vi "Impedance_Single.vi"(0 "Test Params Cluster":T2={"Test Freq. (Hz)"=25000.0, "Output Signal Amplitude\nVolts Pk"=0.1, "Sampling Time (s)"=0.01, "Sampling Rate (Hz)"=250000.0, "Output Channel"="PXI1Slot2/ao1", "Current Channel"="PXI1Slot2/ai1", "Voltage Channel"="PXI1Slot2/ai0", "Trigger Channel"="/PXI1Slot2/ao/StartTrigger", "Number of runs"=5}, 2 "SaveFile?":bool, 5 "LCR Params":T1={"Rg_Vmon"=5000.0, "Rg_Imon"=5000.0, "ESL_Cal"=2.95e-07, "ESR_Cal"=0.0, "Cp_Cal"=0.0, "Rp_Cal"=1000000000.0, "UseCorrection"=TRUE, "R_Shunt"=100.0} {"R_Shunt" format="%#_6p"; "Rg_Vmon" format="%#_6p"; "Rg_Imon" format="%#_6p"; "ESL_Cal" format="%#_6p"; "ESR_Cal" format="%#_6p"; "Cp_Cal" format="%#_6p"; "Rp_Cal" format="%#_6p"}, 12 "File Name String":string="Test", 13 "Path":path=path "C:/Users/MPI/Documents/Test Saving Data", 14 "Experiment Title":string="Experiment Title") -> (4 "Mean Signal\nImpedance cluster":T3={"|Z|"=131.4492234563314, "Phase(Z)"=77.90762243322018, "Re(Z)"=27.537098036686675, "Imag(Z)"=128.53251175866149, "Ls"=0.0008182633837763256, "Cs"=-4.952986319624157e-08, "Rp"=0.0, "Cp"=0.0} {"|Z|" format="%#_6p"; "Phase(Z)" format="%#_6p"; "Re(Z)" format="%#_6p"; "Imag(Z)" format="%#_6p"; "Ls" format="%#_6p"; "Cs" format="%#_6p"; "Rp" format="%#_6p"; "Cp" format="%#_6p"})   [LabVIEW 2020]
uses:
  <vilib>/Analysis/baseanly.llb/Mean (CDB).vi
  <vilib>/Analysis/NI_AALBase.lvlib
panel:
  out "Progress":i32(slide) scale=0.0..100.0
  in  "Tab Control":enum32{"Inputs", "Outputs", "Additional Plots"}(tab)
  out "Impedance (Mag)":dbl=131.44922360893165 format="%_4p"
  out "Impedance (Phase)":dbl=77.90762242326527 format="%_3p"
  out "Inductance":dbl=0.0008182633837921632 format="%#_3p"
  out "Capacitance":dbl=-4.9529863304224986e-08 format="%#_3p"
  out "Real (Z)":dbl=27.53709808707976 format="%#_4p"
  out "St. Dev - |Z|":dbl=0.006733204606830156 format="%.4p"
  out "St. Dev - L":dbl=4.20379350558212e-08 format="%.2p"
  out "St. Dev - C":dbl=2.5446531556775277e-12 format="%.2p"
  out "St. Dev - R":dbl=0.00676584259927313 format="%.2p"
  out "Mag Real Imag":cluster{"mean":dbl, "mean":dbl, "Imag(Z)":dbl}(graph)
  out "Time domain Voltage":waveform(dbl)(graph)={"t0"=timestamp(3724414950.391881 s since 1904-01-01), "dt"=3.999999999999989e-06, "Y"=array[2500 elements], "attributes"=variant("NI_ChannelName"=variant(string "Dev3/ai0"), "NI_UnitDescription"=variant(string "Volts"))}
  out "Time domain Current\n(Measured Voltage)":waveform(dbl)(graph)={"t0"=timestamp(3724414950.478328 s since 1904-01-01), "dt"=3.999999999999989e-06, "Y"=array[2500 elements], "attributes"=variant("NI_ChannelName"=variant(string "Dev3/ai1"), "NI_UnitDescription"=variant(string "Volts"))}
  out "Inductance 2":dbl(graph)
  out "Current Run #":i32=4
  out "Time domain Signals":waveform(dbl)[](graph)=[{"t0"=timestamp(3724414950.391881 s since 1904-01-01), "dt"=3.999999999999989e-06, "Y"=array[2500 elements], "attributes"=variant("NI_ChannelName"=variant(string "Dev3/ai0"), "NI_UnitDescription"=variant(string "Volts"))}, {"t0"=timestamp(3724414950.478328 s since 1904-01-01), "dt"=3.999999999999989e-06, "Y"=array[2500 elements], "attributes"=variant("NI_ChannelName"=variant(string "Dev3/ai1"), "NI_UnitDescription"=variant(string "Volts"))}]
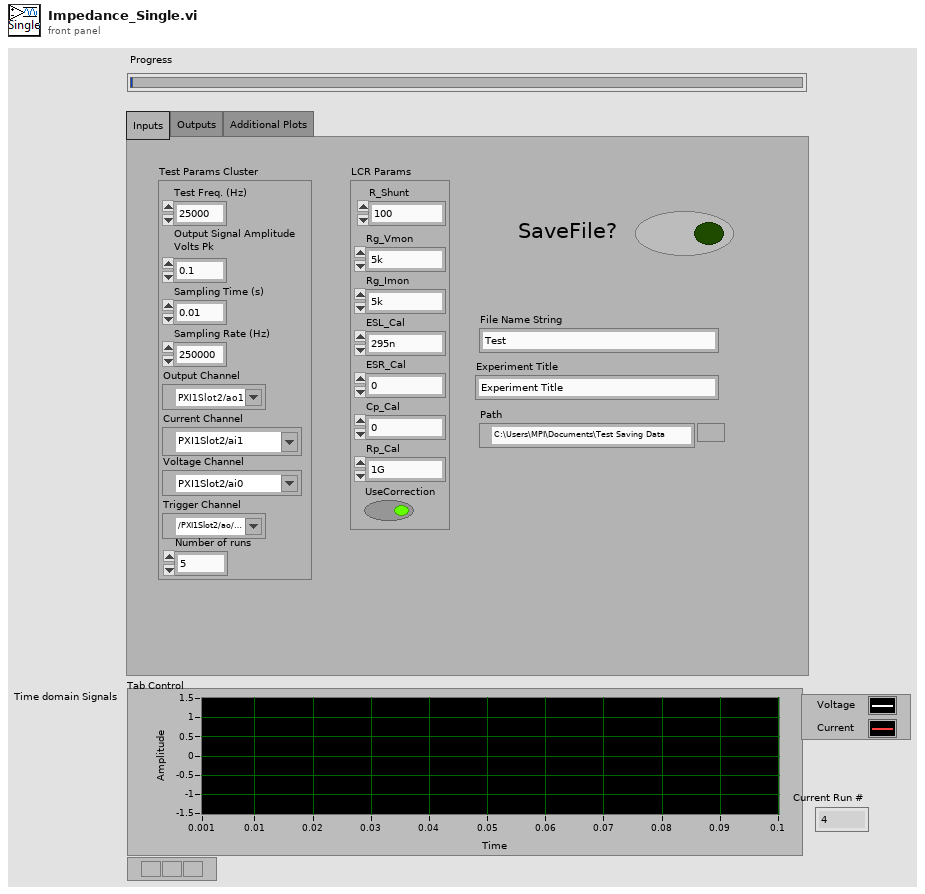
[diagram p1: front panel]
types:
  T1 = cluster{"Rg_Vmon":dbl, "Rg_Imon":dbl, "ESL_Cal":dbl, "ESR_Cal":dbl, "Cp_Cal":dbl, "Rp_Cal":dbl, "UseCorrection":bool, "R_Shunt":dbl}
  T2 = cluster{"Test Freq. (Hz)":dbl, "Output Signal Amplitude\nVolts Pk":dbl, "Sampling Time (s)":dbl, "Sampling Rate (Hz)":dbl, "Output Channel":tag, "Current Channel":tag, "Voltage Channel":tag, "Trigger Channel":tag, "Number of runs":i32}
  T3 = cluster{"|Z|":dbl, "Phase(Z)":dbl, "Re(Z)":dbl, "Imag(Z)":dbl, "Ls":dbl, "Cs":dbl, "Rp":dbl, "Cp":dbl}
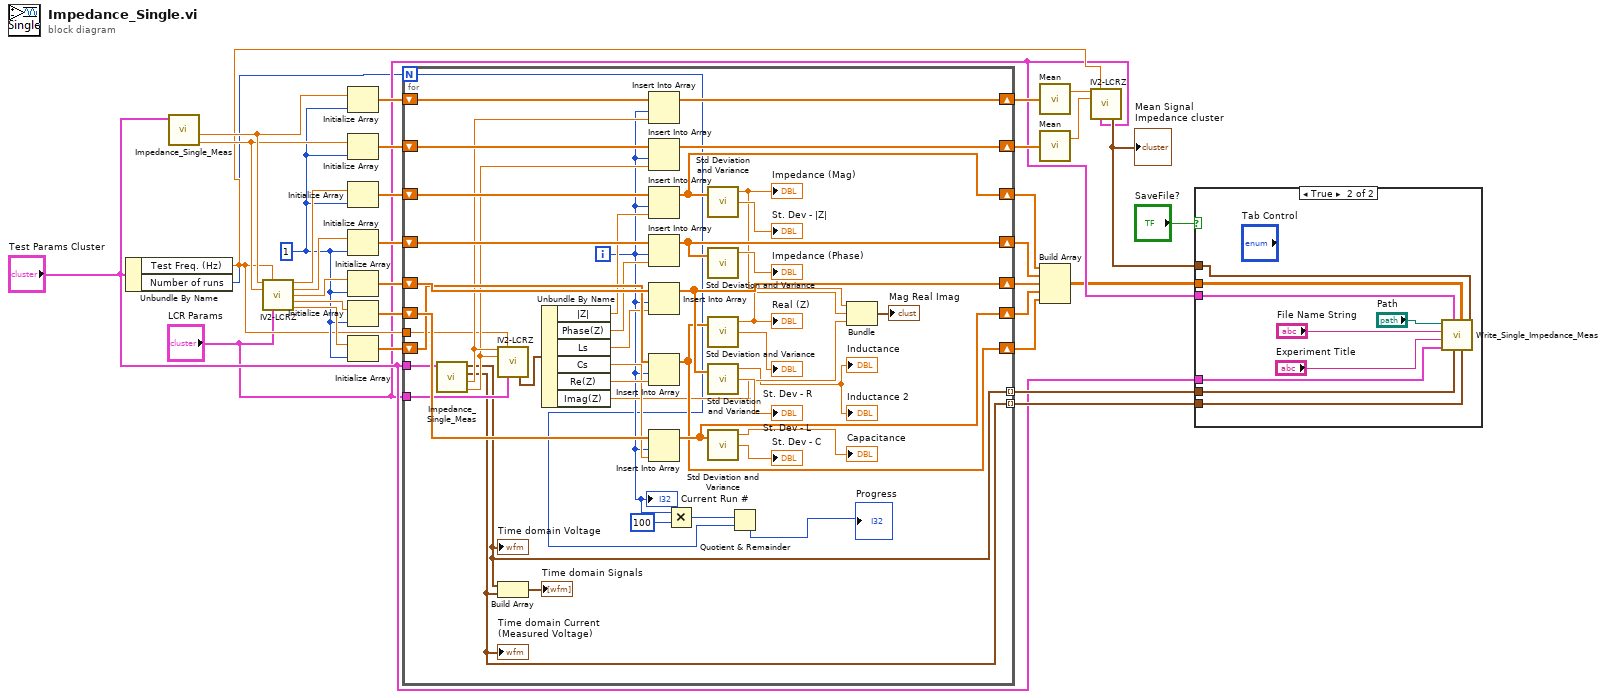
[diagram p0: block diagram]
diagram:
  w21 = 1 ("dimension size")
  n1 = Unbundle By Name("Test Params Cluster") -> ("Test Freq. (Hz)"=w9:dbl, "Number of runs"=w7:i32)
  n2 = call "Impedance_Single_Meas.vi"("Test Params Cluster"="Test Params Cluster") -> ("Current Complex"=w22:cdb, "Voltage Complex"=w23:cdb)  [unwired: 7 in, 2 out]
  n3 = call "IV2-LCRZ.vi"("Voltage In"=w23, "Test Frequency"=w9, "Current In"=w22, "LCR Params"="LCR Params") -> ("Impedance (Mag)"=w31:dbl, "Impedance (Phase)"=w30:dbl, "Ls"=w29:dbl, "Cs"=w28:dbl, "Real (Z)"=w27:dbl)  [unwired: 6 in, 1 out]
  n4 = Initialize Array(w23, w21) -> (w20:cdb[])
  n5 = Initialize Array(w22, w21) -> (w19:cdb[])
  n6 = Initialize Array(w31, w21) -> (w33:dbl[])
  n7 = Initialize Array(w30, w21) -> (w32:dbl[])
  n8 = Initialize Array(w29, w21) -> (w26:dbl[])
  n9 = Initialize Array(w28, w21) -> (w25:dbl[])
  n10 = Initialize Array(w27, w21) -> (w24:dbl[])
  n11 = for {
    N: w7 -> [w34]
    shift-right: [w63] -> w6
    shift-left: w33 -> [w76]
    shift-right: [w62] -> w5
    shift-left: w32 -> [w75]
    shift-right: [w61] -> w4
    shift-left: w26 -> [w74]
    shift-right: [w57] -> w3
    shift-left: w25 -> [w73]
    shift-right: [w55] -> w2
    shift-left: w24 -> [w72]
    shift-right: [w67] -> w18
    shift-left: w20 -> [w71]
    shift-right: [w66] -> w17
    shift-left: w19 -> [w70]
    tunnel: "LCR Params" -> [w54]
    tunnel: "Test Params Cluster" -> [w47]
    tunnel: [w46] -> w12 mode=indexing
    tunnel: [w45] -> w11 mode=indexing
    tunnel: w9 -> [w44]
    i -> [w37]
    n12 = call "Impedance_Single_Meas.vi"("Test Params Cluster"=w47) -> ("Current Complex"=w68:cdb, "Voltage Complex"=w69:cdb, "Time domain Current"=w45:waveform(dbl), "Time domain Voltage"=w46:waveform(dbl))  [unwired: 7 in]
    "Time domain Current\n(Measured Voltage)" <- w45
    "Time domain Voltage" <- w46
    n13 = call "IV2-LCRZ.vi"("Voltage In"=w69, "Test Frequency"=w44, "Current In"=w68, "LCR Params"=w54) -> ("Impedance cluster"=w53:T3)  [unwired: 6 in, 5 out]
    n14 = Build Array(w46, w45) -> (→"Time domain Signals":waveform(dbl)[])
    n15 = Unbundle By Name(w53) -> ("|Z|"=w52:dbl, "Phase(Z)"=w51:dbl, "Ls"=w48:dbl, "Cs"=w49:dbl, "Re(Z)"=w50:dbl, "Imag(Z)"=w40:dbl)
    n16 = Insert Into Array(array=w71, index=w37, new element=w69) -> (w67:cdb[])
    n17 = Insert Into Array(array=w70, index=w37, new element=w68) -> (w66:cdb[])
    n18 = Insert Into Array(array=w76, index=w37, new element=w52) -> (w63:dbl[])
    n19 = Insert Into Array(array=w75, index=w37, new element=w51) -> (w62:dbl[])
    n20 = Insert Into Array(array=w74, index=w37, new element=w48) -> (w61:dbl[])
    n21 = Insert Into Array(array=w72, index=w37, new element=w50) -> (w55:dbl[])
    n22 = Insert Into Array(array=w73, index=w37, new element=w49) -> (w57:dbl[])
    n23 = Multiply(x=w37, y=100) -> (x*y=w35:i32)
    n24 = call <vilib>:"Std Deviation and Variance.vi"("X"=w63) -> ("mean"=w42:dbl, "standard deviation"=→"St. Dev - |Z|":dbl)  [unwired: 1 in, 1 out]
    "Impedance (Mag)" <- w42
    n25 = call <vilib>:"Std Deviation and Variance.vi"("X"=w62) -> ("mean"=→"Impedance (Phase)":dbl)  [unwired: 1 in, 2 out]
    n26 = call <vilib>:"Std Deviation and Variance.vi"("X"=w55) -> ("mean"=w41:dbl, "standard deviation"=→"St. Dev - R":dbl)  [unwired: 1 in, 1 out]
    "Real (Z)" <- w41
    n27 = call <vilib>:"Std Deviation and Variance.vi"("X"=w61) -> ("mean"=→"Inductance" →"Inductance 2":dbl, "standard deviation"=→"St. Dev - L":dbl)  [unwired: 1 in, 1 out]
    n28 = call <vilib>:"Std Deviation and Variance.vi"("X"=w57) -> ("mean"=→"Capacitance":dbl, "standard deviation"=→"St. Dev - C":dbl)  [unwired: 1 in, 1 out]
    n29 = Quotient & Remainder(x=w35, y=w34) -> (floor(x/y)=→"Progress":i32)  [unwired: 1 out]
    n30 = Bundle("mean"=w42, "mean"=w41, "Imag(Z)"=w40) -> (→"Mag Real Imag":cluster{"mean":dbl, "mean":dbl, "Imag(Z)":dbl})  [unwired: 1 in]
    "Current Run #" <- w37
  }
  n31 = call-poly <vilib>:"Mean.vi"("X"=w18) -> ("mean"=w16:cdb)  [unwired: 1 out]
  n32 = call-poly <vilib>:"Mean.vi"("X"=w17) -> ("mean"=w15:cdb)  [unwired: 1 out]
  n33 = Build Array(w6, w5, w4, w3, w2) -> (w1:dbl[][])
  n34 = call "IV2-LCRZ.vi"("Voltage In"=w16, "Test Frequency"=w9, "Current In"=w15, "LCR Params"="LCR Params") -> ("Impedance cluster"=w14:T3)  [unwired: 6 in, 5 out]
  "Mean Signal\nImpedance cluster" <- w14
  n35 = case shown="True" "SaveFile?" {
    tunnel: "Test Params Cluster" -> [_ w83]
    tunnel: w14 -> [_ w82]
    tunnel: "LCR Params" -> [_ w81]
    tunnel: w12 -> [_ w80]
    tunnel: w11 -> [_ w79]
    tunnel: w1 -> [_ w78]
    frame False {
    }
    frame True {
      n36 = call "Write_Single_Impedance_Meas.vi"("Mean Signal\nImpedance cluster"=w82, "Current"=w79, "Run Impedances array"=w78, "Voltage"=w80, "Compensation and Gain"=w81, "Test Params Cluster"=w83, "Experiment Title"="Experiment Title", "File Name String"="File Name String", "Path"="Path") -> ()  [unwired: 3 in]
    }
  }
